vi "495Dashboardv1.vi"() -> ()   [LabVIEW 2020]
panel:
  in  "Tab Control":enum32{"Page 1", "Page 2"}(tab)
  in  "Beam Gain":dbl
  in  "Beam Angle":dbl
  in  "TX Stage Position":dbl(slide) scale=0.0..10.0
  out "XY Graph":cluster{"X":dbl, "Y":dbl}[](graph)
  out "XY Graph 2":cluster{"X":dbl, "Y":dbl}[](graph)
  in  "RX Stage Position":dbl(slide) scale=0.0..10.0
  in  "Beam Angle":dbl
  in  "Beam Gain":dbl
  # "TX mmWave Band"
  # "RX mmWave Band"
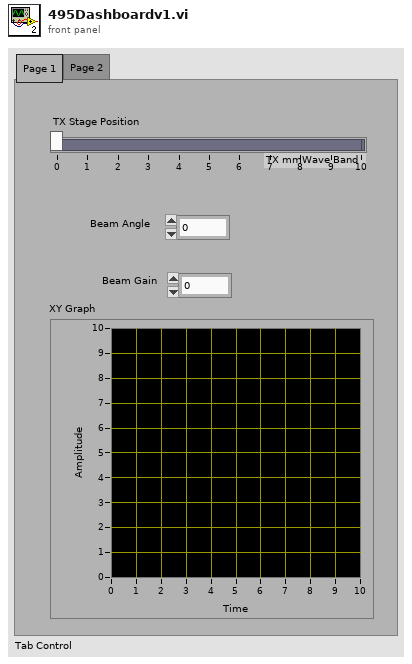
[diagram p1: front panel]
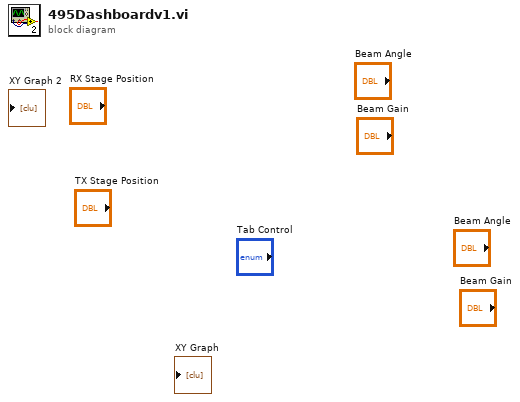
[diagram p0: block diagram]
diagram:
